vi "Get Short Help.vi"(8 "error in (no error)":errorcluster, 11 "Upgrade in":refnum<class "Upgrade.lvclass">) -> (0 "error out":errorcluster, 2 "Short Help":string, 3 "Upgrade out":refnum<class "Upgrade.lvclass">)   [LabVIEW 2020, in "Upgrade.lvlib" / "Upgrade.lvclass"]
uses:
  Upgrade.lvclass
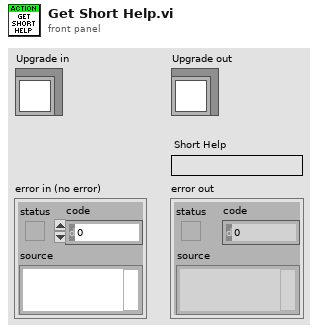
[diagram p1: front panel]
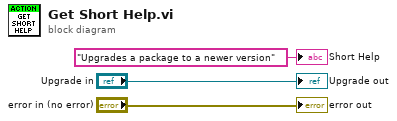
[diagram p0: block diagram]
diagram:
  "error out" <- "error in (no error)"
  "Upgrade out" <- "Upgrade in"
  "Short Help" <- "Upgrades a package to a newer version" ("Short Help")
